vi "8 - Turn Off Lock Panel to Allow Asynchronicity.vi"() -> ()   [LabVIEW 2012]
panel:
  in  "Increment this to 5\nto exit the program":i32
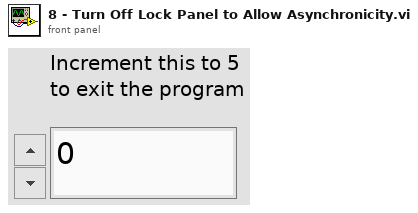
[diagram p1: front panel]
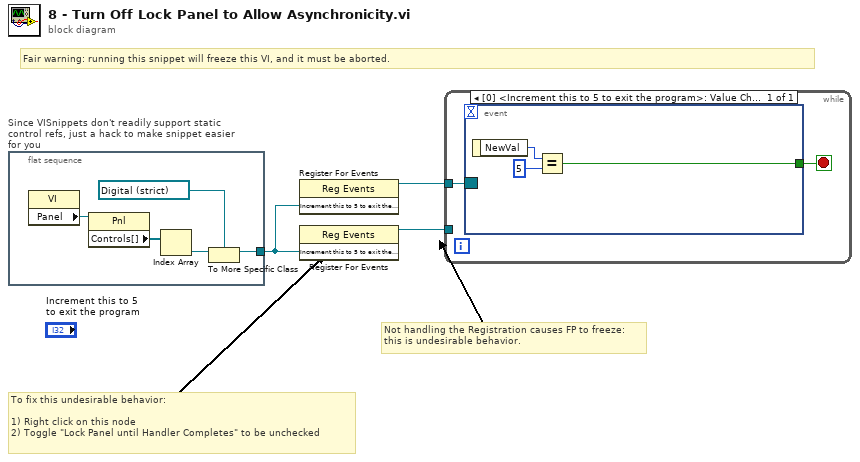
[diagram p0: block diagram]
diagram:
  # "To fix this undesirable behavior:\n\n1) Right click on this node\n2) Toggle \"Lock Panel until Handler Completes\" to be unchecked"
  # "Not handling the Registration causes FP to freeze:\nthis is undesirable behavior."
  # "Fair warning: running this snippet will freeze this VI, and it must be aborted."
  n1 = flat-sequence "Since VISnippets don't readily support static\ncontrol refs, just a hack to make snippet easier for you" {
    tunnel: [w4] -> w1
    frame #0 {
      n2 = property class="VI"() -> ("Panel"=w8:refnum<vi>)  [unwired: 2 in, 2 out]
      n3 = property class="Pnl"(reference=w8) -> ("Controls[]"=w7:refnum<vi>[])  [unwired: 1 in, 2 out]
      n4 = Index Array(array=w7) -> (element=w6:refnum<vi>)  [unwired: 1 in]
      n5 = To More Specific Class(target class=refnum<vi> refnum ("Increment this to 5 to exit the program"), reference=w6) -> (specific class reference=w4:refnum<vi>)  [unwired: 1 in, 1 out]
    }
  }
  n6 = register-events(w1) -> (reference out=w3:refnum<event-registration>)  [unwired: 2 in, 1 out]
  n7 = register-events(w1) -> (reference out=w2:refnum<event-registration>)  [unwired: 2 in, 1 out]
  n8 = while {
    tunnel: w3 -> [w9]
    tunnel: w2 -> [_]
    stop <- w10 stop-if-true
    n9 = event shown="[0] <Increment this to 5 to exit the program>: Value Change" {
      selector: w9 -> [_]
      dyn-events: _ -> [_]
      timeout: _ -> [_]
      tunnel: [w11] -> w10
      event Value Change {
        n10 = event-data() -> ("NewVal"=w13:i32)  [unwired: 1 in]
        n11 = Equal?(x=w13, y=5) -> (x = y?=w11:bool)
      }
    }
  }
